vi "LVClass_WavefrontCorrector Write WavefrontCorrector.vi"(8 "error in (no error)":errorcluster, 10 "WavefrontCorrector":T1, 11 "WavefrontCorrector in":refnum<class "WavefrontCorrector.lvclass">) -> (0 "error out":errorcluster, 3 "WavefrontCorrector out":refnum<class "WavefrontCorrector.lvclass">)   [LabVIEW 2020, in "WavefrontCorrector.lvclass"]
uses:
  WavefrontCorrector.lvclass
  Controls/ClassID.ctl
  Controls/Handle creation.ctl
  WavefrontCorrector.lvclass/WavefrontCorrector.ctl
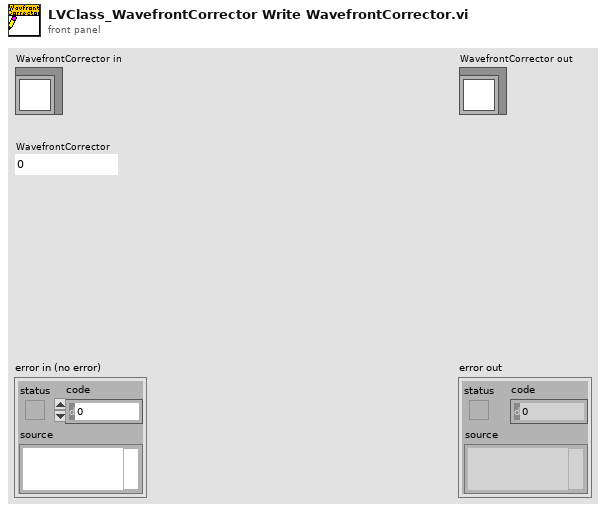
[diagram p1: front panel]
types:
  T1 = typedef "ClassID.ctl" = i64
  T2 = typedef "Handle creation.ctl" = enum16{"By ctor", "By write function"}
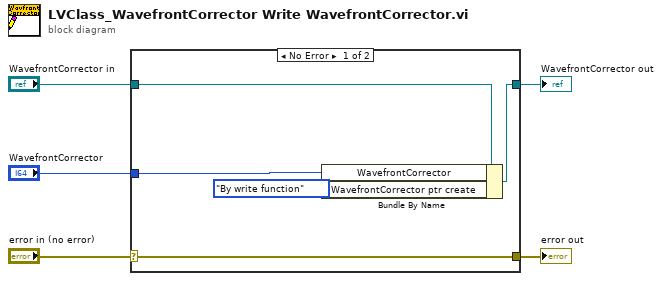
[diagram p0: block diagram]
diagram:
  n1 = case shown="No Error" "error in (no error)" {
    selector: "error in (no error)" -> [w10 w11]
    tunnel: [w10 w11] -> w4
    tunnel: [w8 w12] -> w2
    tunnel: "WavefrontCorrector in" -> [w9 w12]
    tunnel: "WavefrontCorrector" -> [w7 _]
    frame No Error {
      n2 = Bundle By Name(cluster=w9, "WavefrontCorrector"=w7, "WavefrontCorrector ptr create"=Handle_creation."By write function") -> (w8:refnum<class "WavefrontCorrector.lvclass">)
    }
    frame Error {
    }
  }
  "error out" <- w4
  "WavefrontCorrector out" <- w2
